vi "Robot Global Data.vi"() -> ()   [LabVIEW 2012]
doc: "This global VI can contain as many global variables as you need. Place a control on the panel, give it a good name. To read or write to it from a VI, drag the icon to the diagram of that VI. You can also drag from the project. Click on the node to change which global you access. You shouldn't have multiple locations writing to a global or it will cause a race-condition."
panel:
  in  "LShoulderX":dbl
  in  "LHandX":dbl
  in  "LHandY":dbl
  in  "RHipY":dbl
  in  "RHeadY":dbl
  in  "RHandY":dbl
  out "Old iterator":i8
  in  "Enum":enum16{"Default", "Shoot"}(ring)
  in  "turretSpeed":dbl
  out "Auto Align":bool
  out "Align Adjust":dbl
  out "Time Stationary":i32
  out "Time Lined Up":i32
  out "Set Gyro":dbl
  out "Set distance":dbl
  out "Servo":i32
  out "Arm Down":bool
  in  "Arm":enum16{"Up", "Neutral", "Down"}(ring)
  out "Set Shooter speed":dbl
  out "Shooter Offset":dbl
  out "Turret Coarse":dbl
  out "Shooter":dbl
  out "Balance":bool
  out "Shoot":bool
  in  "Bottom":enum16{"Up", "Neutral", "Down"}(ring)
  in  "Middle":enum16{"Up", "Neutral", "Down"}(ring)
  in  "Top":enum16{"Up", "Neutral", "Down"}(ring)
  in  "Lined up?":bool
  in  "Gear":enum16{"Low Gear ", "None", "High Gear"}(ring)
  out "Distance to Target":dbl
  out "Angle to Target":dbl
  out "Top HWA":cluster{dbl, dbl, dbl}
  out "Bottom HWA":cluster{dbl, dbl, dbl}
  out "Right HWA":cluster{dbl, dbl, dbl}
  out "Left HWA":cluster{dbl, dbl, dbl}
  out "Particle Info":T1(array[cluster])
  out "Manual":bool
  out "Turret Speed":dbl
  out "Z axis":dbl
  out "Y axis":dbl
  out "X axis":dbl
  out "Gyro Angle":dbl
  out "Particles":i8
  out "Vision Bottom X":dbl
  out "Target Info":T2(array[cluster])
  in  "LED toggle rate (ms)":u32=20
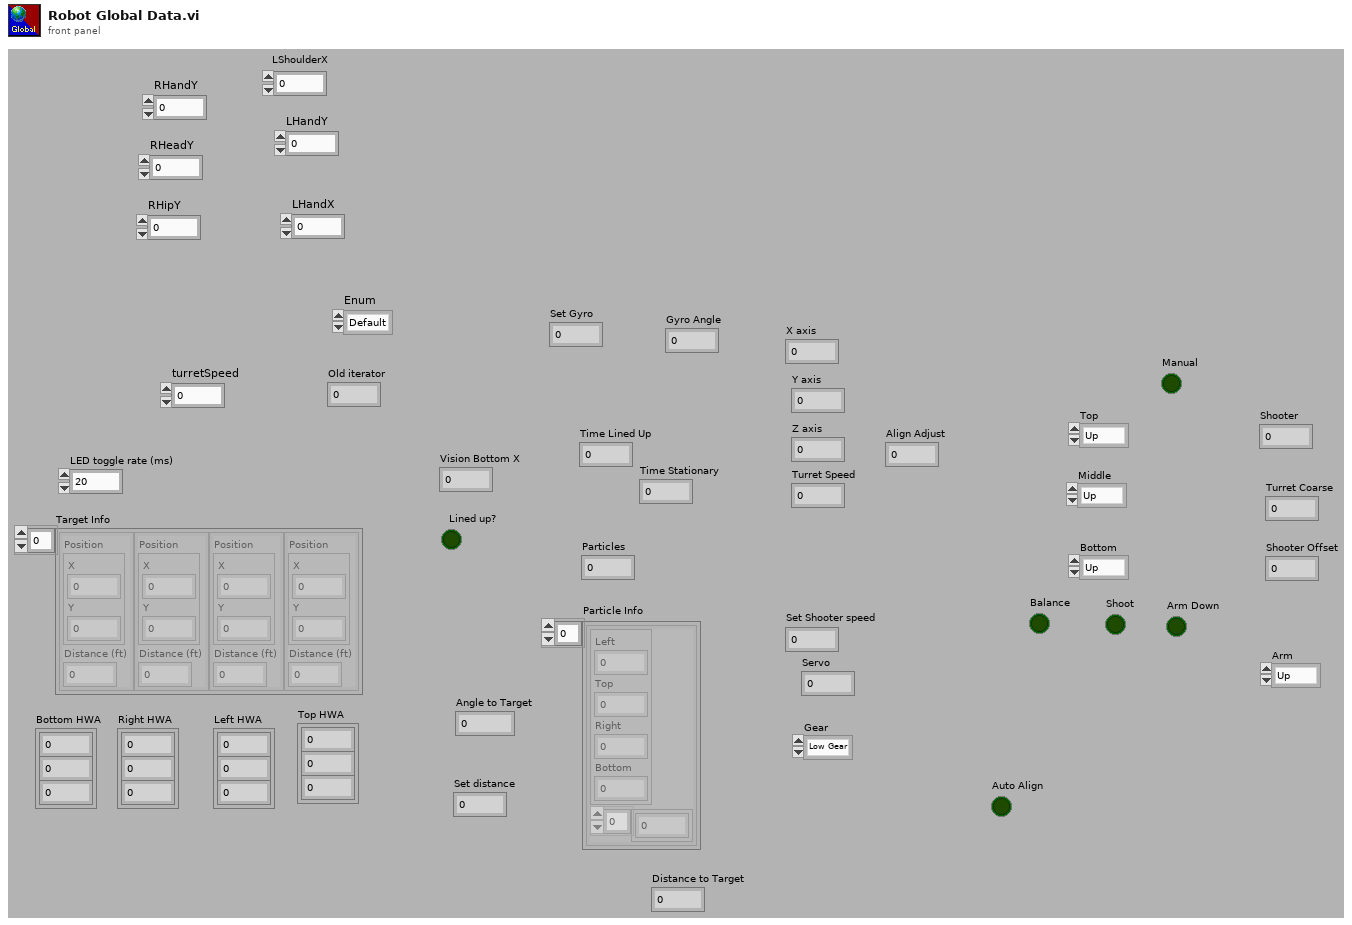
[diagram p1: front panel]
types:
  T1 = cluster{cluster{"Left":dbl, "Top":dbl, "Right":dbl, "Bottom":dbl}, dbl[]}[]
  T2 = cluster{"Position":cluster{"X":dbl, "Y":dbl}, "Distance (ft)":dbl}[]
diagram:
